vi "SEA-9811_ReceiverLoopback_RT.vi"() -> ()   [LabVIEW 2017]
doc: "This example demonstrates the SEA 9811 ARINC-429 receiver loopback mode. This mode is useful for simple receiver tests when no transmitter is available. Please also refer to the FPGA VI.\n\n<B>Prerequisites:</B>\n1. NI CompactRIO\n2. SEA 9811\n\n<B>Instructions:</B>\n1. Run the VI.\n2. Observe that all 8 channels indicate that receiver FIFOs are empty. \n2. Enter data to be written in <B>Rx Sim Data</B> and write it pressing the corresponding button.\n3. Observe that all 8 channels indicate that receiver FIFOs are NOT empty.\n4. Press the button <B>Read Rx Data</B> and notify that all receiver channels return the sent word and the FIFOs become empty.\n5. Press the button <B>Write Rx SimData</B> four times consecutively.\n6. Observe that the receiver FIFOs are full (FIFO depth = 4).\n7. Read the RX data four times to empty the FIFOs again.\n8. Stop the VI.\n\nCopyright (c) 2013-2019 S.E.A. Datentechnik GmbH, Germany"
uses:
  <vilib>/rvi/interface/nirviOpenFPGA/nirviOpenFPGA.xnode
  <vilib>/rvi/interface/nirviReadWriteControl/nirviReadWriteControl.xnode
  <vilib>/rvi/interface/nirviCloseFPGA/nirviCloseFPGA.xnode
  <vilib>/rvi/interface/nirviMethod/nirviMethod.xnode
  SubVIs/SEA-9811_ReceiverLoopback_RCR.ctl
  Projekte/SEA/workspace_9811/cRIO_SEA_9811/Software/.SourceCode/Examples/SEA-9811_ReceiverLoopback/SEA-9811_ReceiverLoopback_FPGA.vi
  <vilib>/rvi/errors/niLvFpgaMergeErrorWithErrorCode.vi
  SubVIs/SEA-9811_ReceiverLoopback_RSR.ctl
panel:
  out "Receiver Status Register (RSR)":T1={"RSR0: FIFO channel 0 empty"=TRUE, "RSR1: FIFO channel 1 empty"=TRUE, "RSR2: FIFO channel 2 empty"=TRUE, "RSR3: FIFO channel 3 empty"=TRUE, "RSR4: FIFO channel 4 empty"=TRUE, "RSR5: FIFO channel 5 empty"=TRUE, "RSR6: FIFO channel 6 empty"=TRUE, "RSR7: FIFO channel 7 empty"=TRUE, "RSR8: FIFO channel 0 full"=FALSE, "RSR9: FIFO channel 1 full"=FALSE, "RSR10: FIFO channel 2 full"=FALSE, "RSR11: FIFO channel 3 full"=FALSE, "RSR12: FIFO channel 4 full"=FALSE, "RSR13: FIFO channel 5 full"=FALSE, "RSR14: FIFO channel 6 full"=FALSE, "RSR15: FIFO channel 7 full"=FALSE}
  out "CH7":u32 format="%08x"
  out "CH6":u32 format="%08x"
  out "CH5":u32 format="%08x"
  out "CH4":u32 format="%08x"
  out "CH3":u32 format="%08x"
  out "CH2":u32 format="%08x"
  out "CH1":u32 format="%08x"
  out "CH0":u32 format="%08x"
  in  "stop":bool
  in  "Rx Sim Data":u32=2271560481 format="%08x"
  in  "Read Rx Data":bool
  in  "Send Rx Sim Data":bool
  # "Please refer to VI description for instructions!"
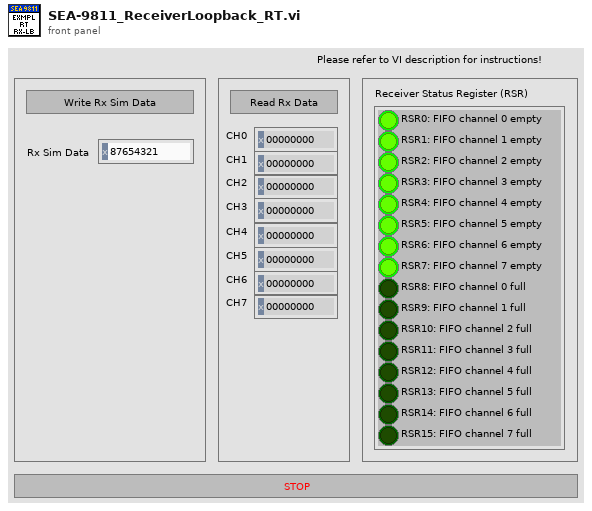
[diagram p1: front panel]
types:
  T1 = typedef "SEA-9811_ReceiverLoopback_RSR.ctl" = cluster{"RSR0: FIFO channel 0 empty":bool, "RSR1: FIFO channel 1 empty":bool, "RSR2: FIFO channel 2 empty":bool, "RSR3: FIFO channel 3 empty":bool, "RSR4: FIFO channel 4 empty":bool, "RSR5: FIFO channel 5 empty":bool, "RSR6: FIFO channel 6 empty":bool, "RSR7: FIFO channel 7 empty":bool, "RSR8: FIFO channel 0 full":bool, "RSR9: FIFO channel 1 full":bool, "RSR10: FIFO channel 2 full":bool, "RSR11: FIFO channel 3 full":bool, "RSR12: FIFO channel 4 full":bool, "RSR13: FIFO channel 5 full":bool, "RSR14: FIFO channel 6 full":bool, "RSR15: FIFO channel 7 full":bool}
  T2 = typedef "SEA-9811_ReceiverLoopback_RCR.ctl" = cluster{"RCR0: Data rate = ARINC 429 High-Speed (0) or Low-Speed (1)":bool, "RCR1: not used":bool, "RCR2: Label recognition for this channel enabled (1) or disabled (0)":bool, "RCR3: Receiver channel disabled (1) or enabled (0)":bool, "RCR4: Odd parity check for this channel enabled (1) or disabled (0":bool, "RCR5: Receiver normal operation (1) or loopback mode (0)":bool, "RCR6: Receiver Decoder disabled (0) or enabled (1) -> ARINC bits 10 and 9 must match RCR7 and RCR8":bool, "RCR7: If receiver decoder is enabled (RCR6=1), the ARINC bit 10 must match this bit":bool, "RCR8: If receiver decoder is enabled (RCR6=1), the ARINC bit 9 must match this bit":bool, "RCR9: Label bit order for this channel non-reversed (1) or reversed (0)":bool, "RCR10: not used":bool, "RCR11: not used":bool, "RCR12: not used":bool, "RCR13: not used":bool, "RCR14: not used":bool, "RCR15: not used":bool}
  T3 = cluster{"Boolean array[0]":bool, "Boolean array[1]":bool, "Boolean array[2]":bool, "Boolean array[3]":bool, "Boolean array[4]":bool, "Boolean array[5]":bool, "Boolean array[6]":bool, "Boolean array[7]":bool, "Boolean array[8]":bool, "Boolean array[9]":bool, "Boolean array[10]":bool, "Boolean array[11]":bool, "Boolean array[12]":bool, "Boolean array[13]":bool, "Boolean array[14]":bool, "Boolean array[15]":bool}
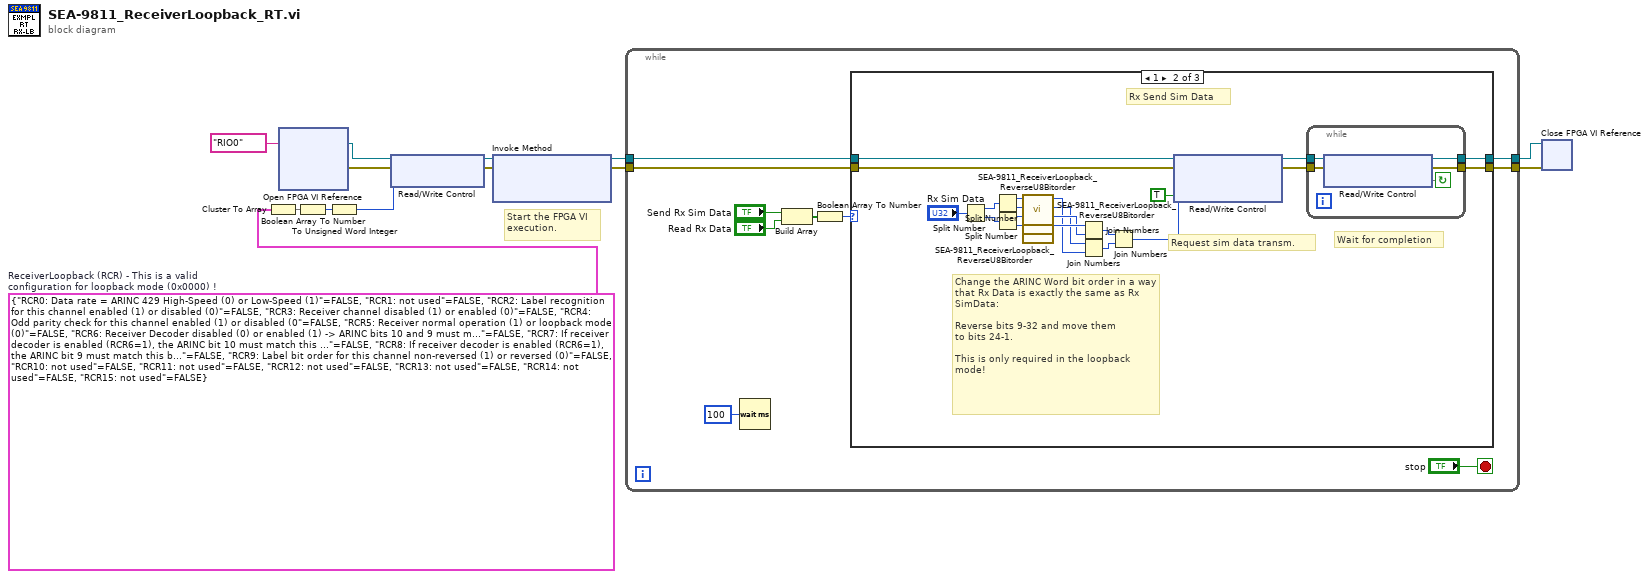
[diagram p0: block diagram]
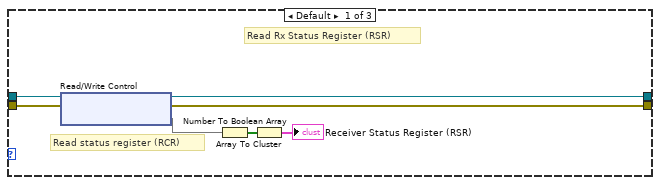
[diagram p2: hidden frame]
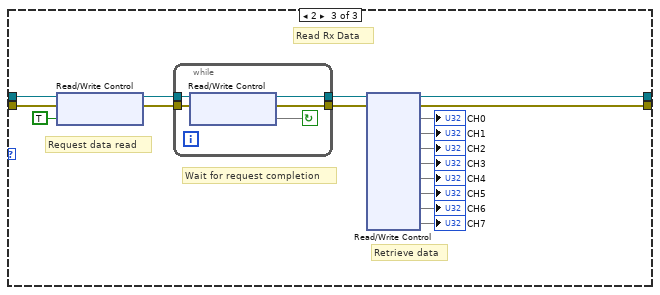
[diagram p3: hidden frame]
diagram:
  w6 = T2 {"RCR0: Data rate = ARINC 429 High-Speed (0) or Low-Speed (1)"=FALSE, "RCR1: not used"=FALSE, "RCR2: Label recognition for this channel enabled (1) or disabled (0)"=FALSE, "RCR3: Receiver channel disabled (1) or enabled (0)"=FALSE, "RCR4: Odd parity check for this channel enabled (1) or disabled (0"=FALSE, "RCR5: Receiver normal operation (1) or loopback mode (0)"=FALSE, "RCR6: Receiver Decoder disabled (0) or enabled (1) -> ARINC bits 10 and 9 must match RCR7 and RCR8"=FALSE, "RCR7: If receiver decoder is enabled (RCR6=1), the ARINC bit 10 must match this bit"=FALSE, "RCR8: If receiver decoder is enabled (RCR6=1), the ARINC bit 9 must match this bit"=FALSE, "RCR9: Label bit order for this channel non-reversed (1) or reversed (0)"=FALSE, "RCR10: not used"=FALSE, "RCR11: not used"=FALSE, "RCR12: not used"=FALSE, "RCR13: not used"=FALSE, "RCR14: not used"=FALSE, "RCR15: not used"=FALSE}  # ReceiverLoopback (RCR) - This is a valid configuration for loopback mode (0x0000) !
  # "Start the FPGA VI\nexecution."
  n1 = Cluster To Array(cluster=w6) -> (array=w5:bool[])
  n2 = xnode "Open FPGA VI Reference"("resource name"=tag "RIO0") -> ("FPGA VI Reference Out"=w2:refnum<k20>, "error out"=w1:errorcluster)  [unwired: 1 in]
  n3 = Boolean Array To Number(Boolean array=w5) -> (number=w4:u32)
  n4 = To Unsigned Word Integer(number=w4) -> (unsigned 16bit integer=w3:u16)
  n5 = xnode "Read/Write Control"("FPGA VI Reference In"=w2, "error in"=w1, "Rx ConfigData"=w3) -> ("FPGA VI Reference Out"=w10:refnum<k20>, "error out"=w8:errorcluster)
  n6 = xnode "Invoke Method"("FPGA VI Reference In"=w10, "error in"=w8) -> ("FPGA VI Reference Out"=w9:refnum<k20>, "error out"=w7:errorcluster)  [unwired: 1 in]
  n7 = while {
    tunnel: w9 -> [w19]
    tunnel: [w18] -> w13
    tunnel: w7 -> [w14]
    tunnel: [w15] -> w11
    stop <- "stop" stop-if-true
    n8 = Wait (ms)(milliseconds to wait=u32 100) -> ()  [unwired: 1 out]
    n9 = Build Array("Send Rx Sim Data", "Read Rx Data") -> (w21:bool[])
    n10 = Boolean Array To Number(Boolean array=w21) -> (number=w20:u32)
    n11 = case shown="1" w20 {
      tunnel: w19 -> [w27 w50 w72]
      tunnel: [w26 w44 w56] -> w18
      tunnel: [w28 w43 w57] -> w15
      tunnel: w14 -> [w29 w42 w70]
      frame Default {
        # "Read status register (RCR)"
        # "Read Rx Status Register (RSR)"
        n12 = xnode "Read/Write Control"("FPGA VI Reference In"=w27, "error in"=w29) -> ("FPGA VI Reference Out"=w26:refnum<k20>, "error out"=w28:errorcluster, "Rx Status Register"=w30)
        n13 = Number To Boolean Array(number=w30) -> (Boolean array=w25:bool[])
        n14 = Array To Cluster(array=w25) -> (cluster=→"Receiver Status Register (RSR)":T3)
      }
      frame 1 {
        # "Request sim data transm."
        # "Wait for completion"
        # "Change the ARINC Word bit order in a way that Rx Data is exactly the same as Rx SimData:\n\nReverse bits 9-32 and move them\nto bits 24-1.\n \nThis is only required in the loopback\nmode!"
        # "Rx Send Sim Data"
        n15 = Split Number(x="Rx Sim Data") -> (hi(x)=w41:u16, lo(x)=w40:u16)
        n16 = Split Number(x=w41) -> (hi(x)=w39:u8, lo(x)=w38:u8)
        n17 = Split Number(x=w40) -> (hi(x)=w37:u8, lo(x)=w36:u8)
        n18 = call "SEA-9811_ReceiverLoopback_ReverseU8Bitorder.vi"("U8 in"=w39) -> ("Bit reversed U8 out"=w32:u8)  [unwired: 10 in]
        n19 = call "SEA-9811_ReceiverLoopback_ReverseU8Bitorder.vi"("U8 in"=w38) -> ("Bit reversed U8 out"=w31:u8)  [unwired: 10 in]
        n20 = call "SEA-9811_ReceiverLoopback_ReverseU8Bitorder.vi"("U8 in"=w37) -> ("Bit reversed U8 out"=w33:u8)  [unwired: 10 in]
        n21 = Join Numbers(hi=w36, lo=w33) -> ((hi.lo)=w35:u16)
        n22 = Join Numbers(hi=w31, lo=w32) -> ((hi.lo)=w34:u16)
        n23 = Join Numbers(hi=w35, lo=w34) -> ((hi.lo)=w49:u32)
        n24 = xnode "Read/Write Control"("FPGA VI Reference In"=w50, "error in"=w42, "Rx Sim Data"=w49, "Write Rx SimData"=TRUE ("Write SimData")) -> ("FPGA VI Reference Out"=w46:refnum<k20>, "error out"=w45:errorcluster)
        n25 = while {
          tunnel: [w54] -> w43
          tunnel: [w53] -> w44
          tunnel: w45 -> [w52]
          tunnel: w46 -> [w51]
          stop <- w55 continue-if-true
          n26 = xnode "Read/Write Control"("FPGA VI Reference In"=w51, "error in"=w52) -> ("FPGA VI Reference Out"=w53:refnum<k20>, "error out"=w54:errorcluster, "Write Rx SimData"=w55)
        }
      }
      frame 2 {
        # "Retrieve data"
        # "Wait for request completion"
        # "Request data read"
        # "Read Rx Data"
        n27 = xnode "Read/Write Control"("FPGA VI Reference In"=w72, "error in"=w70, "Read Rx Data"=TRUE ("Command Finished")) -> ("FPGA VI Reference Out"=w69:refnum<k20>, "error out"=w68:errorcluster)
        n28 = while {
          tunnel: [w76] -> w59
          tunnel: [w75] -> w58
          tunnel: w68 -> [w74]
          tunnel: w69 -> [w73]
          stop <- w77 continue-if-true
          n29 = xnode "Read/Write Control"("FPGA VI Reference In"=w73, "error in"=w74) -> ("FPGA VI Reference Out"=w75:refnum<k20>, "error out"=w76:errorcluster, "Read Rx Data"=w77)
        }
        n30 = xnode "Read/Write Control"("FPGA VI Reference In"=w58, "error in"=w59) -> ("FPGA VI Reference Out"=w56:refnum<k20>, "error out"=w57:errorcluster, "CH0"=→"CH0", "CH1"=→"CH1", "CH2"=→"CH2", "CH3"=→"CH3", "CH4"=→"CH4", "CH5"=→"CH5", "CH6"=→"CH6", "CH7"=→"CH7")
      }
    }
  }
  n31 = xnode "Close FPGA VI Reference"("FPGA VI Reference In"=w13, "error in"=w11) -> ()  [unwired: 1 out]
